vi "Create Recipe.vi"(10 "RecipeCreate inputs":T2, 11 "Refnum in":T1) -> ()   [LabVIEW 2024]
uses:
  CTRLS/RecipeCreate inputs.ctl
  <vilib>/addons/database/Connection.llb/Conn ObjectReference.ctl
  CTRLS/DB operation Selector.ctl
  <vilib>/addons/database/NI_Database_API.lvlib
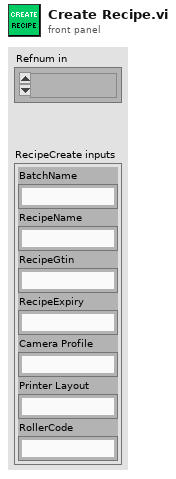
[diagram p1: front panel]
types:
  T1 = typedef "NI_Database_API.lvlib/Conn ObjectReference.ctl" = refnum<k1>
  T2 = typedef "RecipeCreate inputs.ctl" = cluster{"BatchName":string, "RecipeName":string, "RecipeGtin":string, "RecipeExpiry":string, "Camera Profile":string, "Printer Layout":string, "RollerCode":string}
  T3 = typedef "DB operation Selector.ctl" = enum16{"Select", "Insert", "Update", "Execute select Query", "Execute update query"}
  T4 = cluster{string, "RecipeName":string, "RecipeGtin":string, "RecipeExpiry":string, string, string, "RollerCode":string}
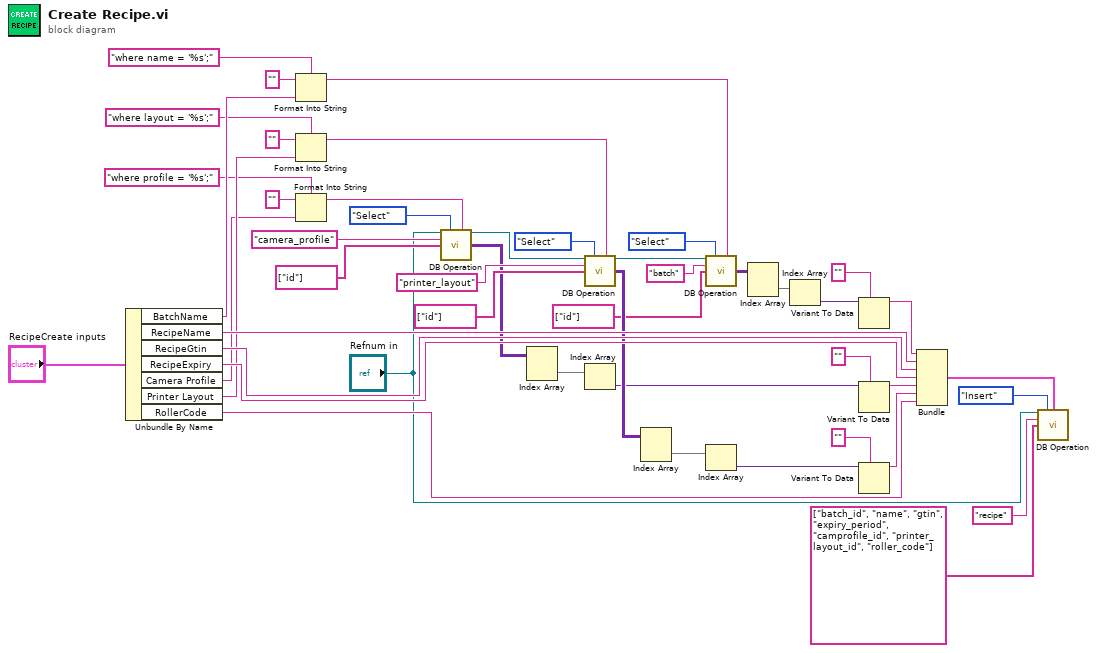
[diagram p0: block diagram]
diagram:
  n1 = Unbundle By Name("RecipeCreate inputs") -> ("BatchName"=w32:string, "RecipeName"=w43:string, "RecipeGtin"=w44:string, "RecipeExpiry"=w45:string, "Camera Profile"=w24:string, "Printer Layout"=w25:string, "RollerCode"=w48:string)
  n2 = Format Into String(format string="where name = '%s';" ("Condition"), initial string="", w32) -> (resulting string=w33:string)  [unwired: 1 in, 1 out]
  n3 = Format Into String(format string="where layout = '%s';" ("Condition"), initial string="", w25) -> (resulting string=w19:string)  [unwired: 1 in, 1 out]
  n4 = Format Into String(format string="where profile = '%s';" ("Condition"), initial string="", w24) -> (resulting string=w9:string)  [unwired: 1 in, 1 out]
  n5 = call "DB Operation.vi"("connection reference"="Refnum in", "DB Op Selector"=DB_operation_Selector."Select", "Condition"=w9, "table"="camera_profile", "columns"=string[] ["id"]) -> ("connection reference out"=w23:T1, "data out"=w12:variant[][])  [unwired: 8 in, 1 out]
  n6 = Index Array(array=w12) -> (element=w13:variant[])  [unwired: 2 in]
  n7 = call "DB Operation.vi"("connection reference"=w23, "DB Op Selector"=DB_operation_Selector."Select", "Condition"=w19, "table"="printer_layout", "columns"=string[] ["id"]) -> ("connection reference out"=w29:T1, "data out"=w34:variant[][])  [unwired: 8 in, 1 out]
  n8 = Index Array(array=w13) -> (element=w14:variant)  [unwired: 1 in]
  n9 = Index Array(array=w34) -> (element=w35:variant[])  [unwired: 2 in]
  n10 = call "DB Operation.vi"("connection reference"=w29, "DB Op Selector"=DB_operation_Selector."Select", "Condition"=w33, "table"="batch", "columns"=string[] ["id"]) -> ("data out"=w41:variant[][])  [unwired: 8 in, 2 out]
  n11 = Index Array(array=w35) -> (element=w36:variant)  [unwired: 1 in]
  n12 = Index Array(array=w41) -> (element=w38:variant[])  [unwired: 2 in]
  n13 = Index Array(array=w38) -> (element=w39:variant)  [unwired: 1 in]
  n14 = Variant To Data(type="", Variant=w39) -> (data=w42:string)  [unwired: 1 in, 1 out]
  n15 = Variant To Data(type="", Variant=w14) -> (data=w46:string)  [unwired: 1 in, 1 out]
  n16 = Variant To Data(type="", Variant=w36) -> (data=w47:string)  [unwired: 1 in, 1 out]
  n17 = Bundle(w42, "RecipeName"=w43, "RecipeGtin"=w44, "RecipeExpiry"=w45, w46, w47, "RollerCode"=w48) -> (w1:T4)  [unwired: 1 in]
  n18 = call "DB Operation.vi"("connection reference"="Refnum in", "DB Op Selector"=DB_operation_Selector."Insert", "data"=w1, "table"="recipe", "columns"=string[] ["batch_id", "name", "gtin", "expiry_period", "camprofile_id", "printer_layout_id", "roller_code"]) -> ()  [unwired: 8 in, 3 out]
